vi "motorJoystickcore2.vi"(4 "button info":T2, 5 "dir":dbl[](array[numeric]), 6 "axis info":T1, 7 "Motor settings (X,Y)":cluster{"Vmax (mm/s)":sgl, "Acc (mm/s/s)":sgl}={"Vmax (mm/s)"=0.1, "Acc (mm/s/s)"=0.05}, 8 "error in":errorcluster[](array[cluster]), 9 "Motor Limits":T3, 10 "Array in":refnum<k7>[](array[refnum])) -> (0 "error out":errorcluster[](array[cluster]), 1 "dir 2":dbl[](array[numeric]), 2 "XYZ position":sgl[](array[numeric]))   [LabVIEW 2014]
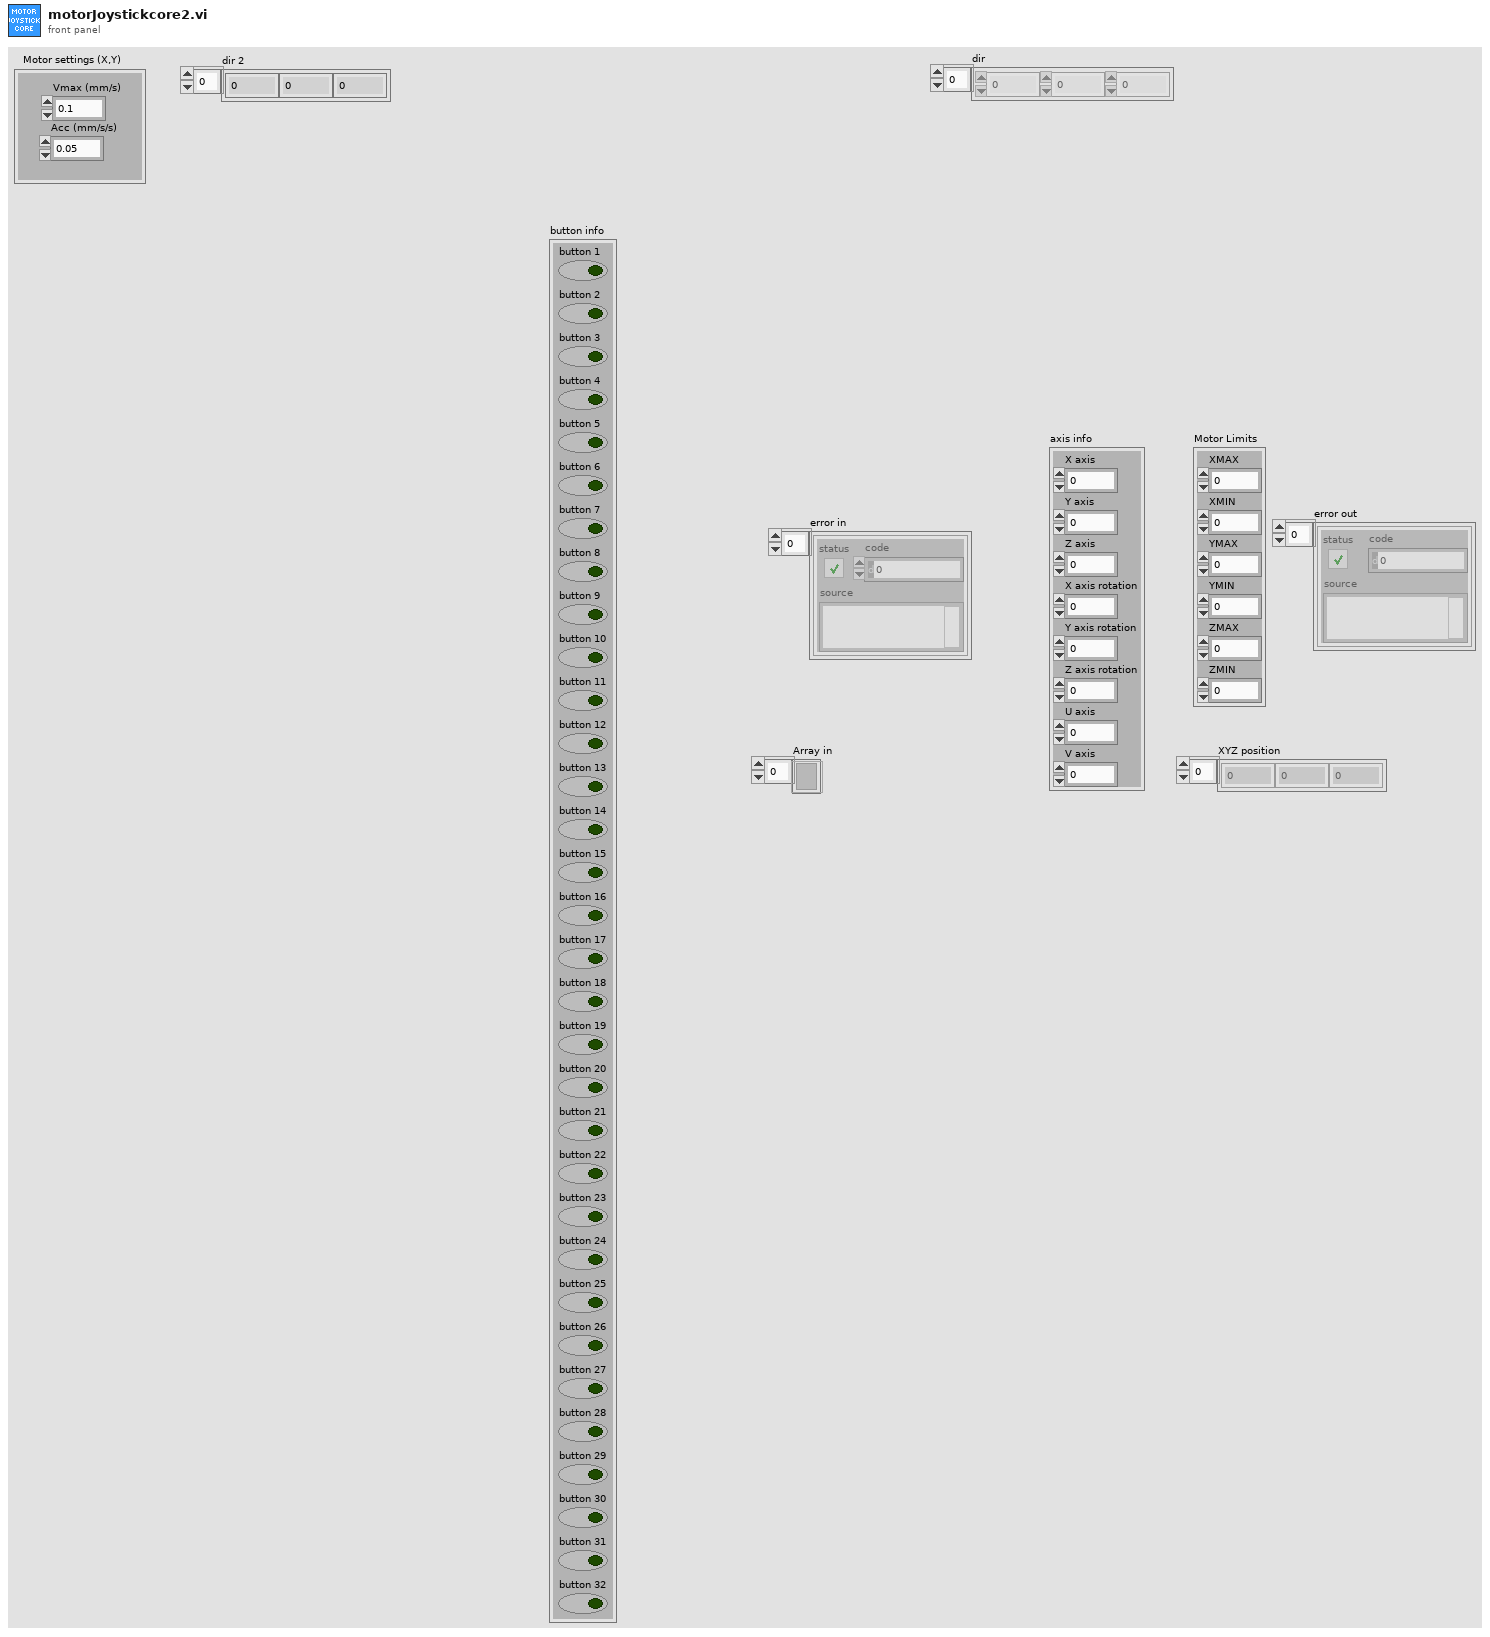
[diagram p1: front panel]
types:
  T1 = cluster{"X axis":i32, "Y axis":i32, "Z axis":i32, "X axis rotation":i32, "Y axis rotation":i32, "Z axis rotation":i32, "U axis":i32, "V axis":i32}
  T2 = cluster{"button 1":bool, "button 2":bool, "button 3":bool, "button 4":bool, "button 5":bool, "button 6":bool, "button 7":bool, "button 8":bool, "button 9":bool, "button 10":bool, "button 11":bool, "button 12":bool, "button 13":bool, "button 14":bool, "button 15":bool, "button 16":bool, "button 17":bool, "button 18":bool, "button 19":bool, "button 20":bool, "button 21":bool, "button 22":bool, "button 23":bool, "button 24":bool, "button 25":bool, "button 26":bool, "button 27":bool, "button 28":bool, "button 29":bool, "button 30":bool, "button 31":bool, "button 32":bool}
  T3 = cluster{"XMAX":sgl, "XMIN":sgl, "YMAX":sgl, "YMIN":sgl, "ZMAX":sgl, "ZMIN":sgl}
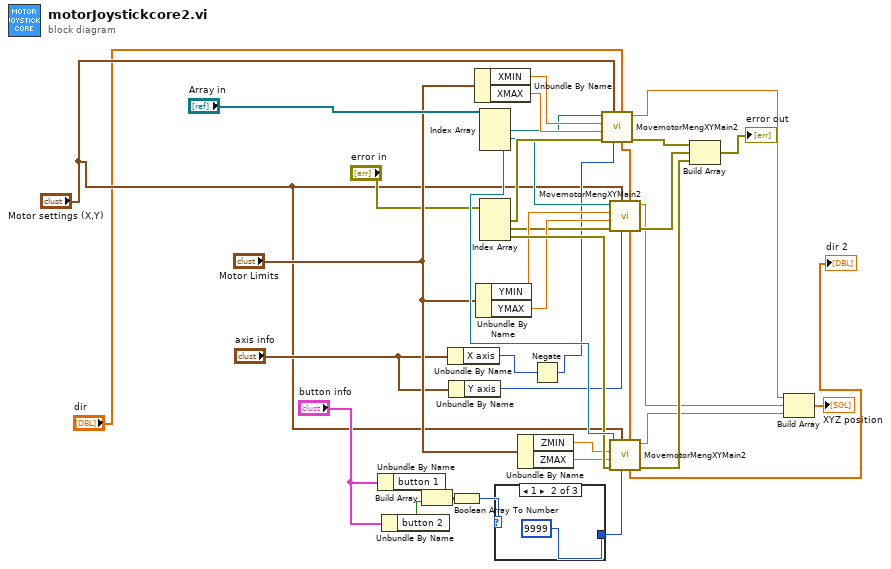
[diagram p0: block diagram]
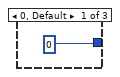
[diagram p2: hidden frame]
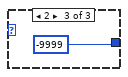
[diagram p3: hidden frame]
diagram:
  n1 = Unbundle By Name("button info") -> ("button 1"=w14:bool)
  n2 = Unbundle By Name("button info") -> ("button 2"=w15:bool)
  n3 = Build Array(w14, w15) -> (w16:bool[])
  n4 = Unbundle By Name("axis info") -> ("X axis"=w7:i32)
  n5 = Unbundle By Name("axis info") -> ("Y axis"=w13:i32)
  n6 = Boolean Array To Number(Boolean array=w16) -> (number=w17:u32)
  n7 = Unbundle By Name("Motor Limits") -> ("XMIN"=w27:sgl, "XMAX"=w28:sgl)
  n8 = Unbundle By Name("Motor Limits") -> ("YMIN"=w29:sgl, "YMAX"=w30:sgl)
  n9 = Index Array(array="Array in") -> (element #1=w19:refnum<k7>, element #2=w20:refnum<k7>, element #3=w38:refnum<k7>)  [unwired: 3 in]
  n10 = Index Array(array="error in") -> (element #1=w22:errorcluster, element #2=w23:errorcluster, element #3=w35:errorcluster)  [unwired: 3 in]
  n11 = case shown="1" w17 {
    tunnel: [0 ("Y axis") 9999 ("Y axis") -9999 ("Y axis")] -> w18
    frame 0, Default {
    }
    frame 1 {
    }
    frame 2 {
    }
  }
  n12 = Unbundle By Name("Motor Limits") -> ("ZMIN"=w31:sgl, "ZMAX"=w32:sgl)
  n13 = Negate(x=w7) -> (-x=w6:i32)
  n14 = call "MovemotorMengXYMain2.vi"("dir"="dir", "Joystick axis"=w6, "Motor settings (X,Y)"="Motor settings (X,Y)", "error in (no error)"=w22, "XorYMAX"=w28, "XorYMIN"=w27, "Automation Refnum in"=w19) -> ("error out"=w24:errorcluster, "XorYPosition"=w11:sgl, "dir 2"=w3:dbl[])  [unwired: 1 in, 1 out]
  n15 = call "MovemotorMengXYMain2.vi"("dir"=w3, "Joystick axis"=w13, "Motor settings (X,Y)"="Motor settings (X,Y)", "error in (no error)"=w23, "XorYMAX"=w30, "XorYMIN"=w29, "Automation Refnum in"=w20) -> ("error out"=w25:errorcluster, "XorYPosition"=w10:sgl, "dir 2"=w2:dbl[])  [unwired: 1 in, 1 out]
  n16 = call "MovemotorMengXYMain2.vi"("dir"=w2, "Joystick axis"=w18, "Motor settings (X,Y)"="Motor settings (X,Y)", "error in (no error)"=w35, "XorYMAX"=w32, "XorYMIN"=w31, "Automation Refnum in"=w38) -> ("error out"=w36:errorcluster, "XorYPosition"=w9:sgl, "dir 2"=→"dir 2":dbl[])  [unwired: 1 in, 1 out]
  n17 = Build Array(w24, w25, w36) -> (→"error out":errorcluster[])
  n18 = Build Array(w11, w10, w9) -> (→"XYZ position":sgl[])
